vi "Initialize.vi"(8 "error in":errorcluster, 11 "Custom Device Item Ref":T1=18446744073709551615 format="%.0x") -> (0 "error out":errorcluster, 3 "Plugin Framework out":refnum<class "Plugin Framework.lvclass">)   [LabVIEW 2024, in "Plugin Framework.lvclass"]
uses:
  Plugin Framework.lvclass
  <vilib>/NI VeriStand/Custom Device API/Custom Device Item Ref.ctl
  Plugin Framework.lvclass/Plugin Framework.ctl
  VS Engine Abstraction/VS Engine/VS Engine.lvclass
  Plugin/Plugin.lvclass
  <vilib>/NI VeriStand/Custom Device API/Custom Device API.lvlib
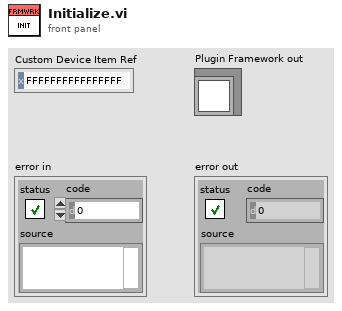
[diagram p1: front panel]
types:
  T1 = typedef "Custom Device API.lvlib/Custom Device Item Ref.ctl" = u64
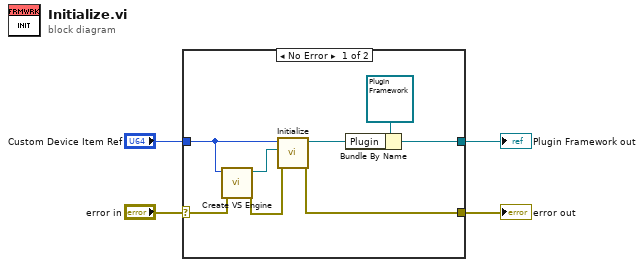
[diagram p0: block diagram]
diagram:
  n1 = case shown="No Error" "error in" {
    selector: "error in" -> [w6 w13]
    tunnel: [w12 w13] -> w3
    tunnel: [w10 _] -> w2
    tunnel: "Custom Device Item Ref" -> [w7 _]
    frame No Error {
      n2 = call "Create VS Engine.vi"("error in"=w6, "Custom Device Item Ref"=w7) -> ("error out"=w5:errorcluster, "VS Engine out"=w8:refnum<class "VS Engine.lvclass">)  [unwired: 8 in]
      n3 = call "Initialize.vi"("error in"=w5, "VS Engine Interface"=w8, "Custom Device Item Ref"=w7) -> ("error out"=w12:errorcluster, "Plugin out"=w9:refnum<class "Plugin.lvclass">)  [unwired: 7 in]
      n4 = Bundle By Name(cluster=refnum<class "Plugin Framework.lvclass"> refnum ("Plugin Framework in"), "Plugin"=w9) -> (w10:refnum<class "Plugin Framework.lvclass">)
    }
    frame Error {
    }
  }
  "error out" <- w3
  "Plugin Framework out" <- w2
